vi "NoiseLoop.vi"(8 "error in (no error)":errorcluster, 11 "Queue in":refnum<queue>) -> (0 "error out":errorcluster)   [LabVIEW 2018]
uses:
  Controls/Enums/NoiseQueueElements.ctl
  Controls/Clusts/Noise_Loop_Clust.ctl
  Controls/Clusts/FPGA_Config_Clust.ctl
  Controls/Enums/TargetNumber.ctl
  Controls/Clusts/Config_Clust.ctl
  Controls/Clusts/UserConfig.ctl
  Controls/PathsCluster.ctl
  Controls/Clusts/FrontPanel_UserConfig.ctl
  Controls/Clusts/Inclinometer_User_Cfg.ctl
  Controls/Clusts/FP_UserTargetConfig.ctl
  Controls/Clusts/FreqShift.ctl
  Controls/Clusts/FPGA_Scale.ctl
  Controls/Enums/ScaleMeasure.ctl
  Controls/RadioButtons/FilterEnableRadio.ctl
  Controls/Clusts/AllNoiseData.ctl
  Controls/Clusts/NoiseFloorData.ctl
  Controls/Clusts/Noise_Targets_Initialized.ctl
  Controls/Clusts/FPGA_Probes.ctl
  Controls/Enums/FP_Loop_Enum.ctl
  Controls/Enums/LogLoopEnum.ctl
  HDF5/HDF5_NoiseInfoClust.ctl
  Controls/Enums/WatchdogTimer_Enum.ctl
  <vilib>/Utility/error.llb/Error Cluster From Error Code.vi
  <vilib>/rvi/errors/niLvFpgaAdjustHostInterfaceError.vi
  <vilib>/rvi/interface/nirviMethod/nirviMethod.xnode
  <vilib>/rvi/interface/nirviReadWriteControl/nirviReadWriteControl.xnode
  <vilib>/FPGAPlugInAG/Dynamic/niLvFpga_StartFifo_Dynamic.vi
  <vilib>/rvi/errors/niLvFpgaMergeErrorWithErrorCode.vi
  <vilib>/FPGAPlugInAG/Dynamic/niLvFpga_ReadFifo_Dynamic.vi
  NiFpgaLv.dll
  <vilib>/rvi/interface/Simulation/niFpgaSimulationCallBeginRW.vi
panel:
  out "Elapsed":u32
  out "NoiseLoopCount":i32
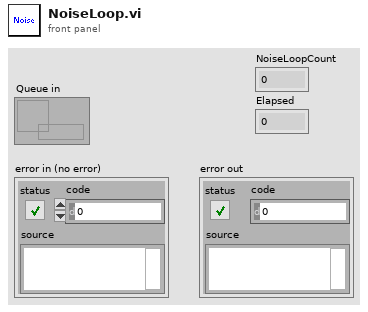
[diagram p1: front panel]
types:
  T1 = typedef "Noise_Loop_Clust.ctl" = cluster{"FPGA":T2, "Config":T4, "AllNoise":T14, "Init'd":T16}
  T2 = typedef "FPGA_Config_Clust.ctl" = cluster{"Target":T3, "Channel":T3, "Ref1":refnum<k20>, "Ref2":refnum<k20>}
  T3 = typedef "TargetNumber.ctl" = enum16{"1", "2", "3", "4"}
  T4 = typedef "Config_Clust.ctl" = cluster{"UsrCfg":T5, "FP_User":T7}
  T5 = typedef "UserConfig.ctl" = cluster{"Paths":T6, "SampleRate":dbl}
  T6 = typedef "PathsCluster.ctl" = cluster{"CfgFile":path, "LogFolder":path, "LogFile":path, "NAS path":path, "ThreshFile":path, "RedunFolder":path}
  T7 = typedef "FrontPanel_UserConfig.ctl" = cluster{"#NoiseSums":u32, "Max_df":u32, "AvgAvg":bool, "#Avg":u16, "AutoCenter":bool, "Inclin":T8, "1":T9, "2":T9, "3":T9, "4":T9, "Target to Probe":T3, "SNR_Thresh":dbl, "Paths":T6, "Connex_Location":string, "SimulateFPGA":bool, "Deadband":dbl}
  T8 = typedef "Inclinometer_User_Cfg.ctl" = cluster{"Vmin":dbl, "Vmax":dbl, "Angle_min":dbl, "Angle_max":dbl, "Offset":dbl, "Pos_Neg":bool}
  T9 = typedef "FP_UserTargetConfig.ctl" = cluster{"Cal_":T10, "Beac":T10, "Scale":T11, "Offset":fxp<+/-,16,16>, "Scale_Noise":fxp<+/-,30,30>, "Scale_Step1":fxp<+/-,17,17>, "Scale_In_RT":ext, "ScaleMeas":fxp<+/-,16,1>, "FreqsToRemove":i32[], "Width":i32[], "ScaleMeasEnum":T12, "FilterEnab":T13}
  T10 = typedef "FreqShift.ctl" = cluster{"Fine":dbl, "Coarse_":dbl}
  T11 = typedef "FPGA_Scale.ctl" = cluster{"Step4":fxp<+/-,23,23>, "Step5":fxp<+/-,23,23>, "Step6":fxp<+/-,23,23>, "Step7":fxp<+/-,23,23>}
  T12 = typedef "ScaleMeasure.ctl" = enum16{"1", "10", "50", "42"}
  T13 = typedef "FilterEnableRadio.ctl" = enum32{"None", "Step 1", "Frequency Shift", "Step 4", "Step 5", "Step 6", "Step 7"}
  T14 = typedef "AllNoiseData.ctl" = cluster{"1":T15, "2":T15, "3":T15, "4":T15}
  T15 = typedef "NoiseFloorData.ctl" = cluster{"df":dbl, "AvgAvgSpectrum":dbl[], "FFT_Index":i32[], "Avg'd":dbl[], "Sum":dbl, "SumdSpectrum":dbl[], "SumCount":u32, "DayOfYear":i32}
  T16 = typedef "Noise_Targets_Initialized.ctl" = cluster{"1":bool, "2":bool, "3":bool, "4":bool}
  T17 = typedef "NoiseQueueElements.ctl" = enum16{"Noise_Startup", "Noise_Init", "Noise_Macro", "Noise_Config", "Noise_NewData", "Noise_Transform", "Noise_SumdTrace", "Noise_Send", "Noise_Probes", "Noise_Exit"}
  T18 = typedef "FPGA_Probes.ctl" = cluster{"Probe 1":i16, "Probe 2":fxp<+/-,16,16>, "Probe 3":fxp<+/-,39,24>, "Probe 4":fxp<+/-,39,24>, "Probe 5":fxp<+/-,16,2>, "Probe 6":fxp<+/-,33,19>, "Probe 7":fxp<+/-,18,1>, "Probe 7_1":fxp<+/-,18,1>, "IProbe":cluster{"Probe 8":fxp<+/-,18,1>, "Probe 9":fxp<+/-,24,1>, "Probe 10":fxp<+/-,24,1>, "Probe 11":fxp<+/-,24,1>, "Probe 12":fxp<+/-,47,24>, "Probe 13":fxp<+/-,24,1>, "Probe 14":fxp<+/-,25,2>, "Probe 15":fxp<+/-,48,25>, "Probe 16":fxp<+/-,24,1>, "Probe 17":fxp<+/-,25,2>, "Probe 18":fxp<+/-,48,25>, "Probe 19":fxp<+/-,24,1>, "Probe20":fxp<+/-,24,1>}, "Probe 21":fxp<+/-,24,5>, "Probe 22":fxp<+/-,54,35>, "Probe 23":fxp<+/-,54,1>, "Probe 24":fxp<+/-,16,1>, "Probe Offsetd":fxp<+/-,16,16>, "CalShiftProbe":fxp<+/-,48,0>, "QProbe":cluster{"Probe 8":fxp<+/-,18,1>, "Probe 9":fxp<+/-,24,1>, "Probe 10":fxp<+/-,24,1>, "Probe 11":fxp<+/-,24,1>, "Probe 12":fxp<+/-,47,24>, "Probe 13":fxp<+/-,24,1>, "Probe 14":fxp<+/-,25,2>, "Probe 15":fxp<+/-,48,25>, "Probe 16":fxp<+/-,24,1>, "Probe 17":fxp<+/-,25,2>, "Probe 18":fxp<+/-,48,25>, "Probe 19":fxp<+/-,24,1>, "Probe20":fxp<+/-,24,1>}, "AI_Over":bool, "10MHzLocked":bool}
  T19 = typedef "LogLoopEnum.ctl" = enum16{"Log_Init", "Log_Config", "Log_CfgAlarm", "Log_TimeDomain", "Log_Tone", "Log_NoiseTrace", "Log_NoiseSum", "Log_DO", "Log_AI", "Log_TC", "Log_Disdrom", "Log_Weather", "Log_TE", "Log_ADAM", "Log_UPS", "Log_ChkTime", "Log_Alarm", "Log_SSH", "Log_Write", "Log_Exit"}
  T20 = typedef "WatchdogTimer_Enum.ctl" = enum16{"ResetAll", "CheckAll", "HW1", "HW2", "Tones", "FP", "Noise", "Log", "TCP", "AI", "TC", "ADAM", "Disdrom", "TE", "Weather"}
  T21 = typedef "HDF5_NoiseInfoClust.ctl" = cluster{"Timestring":string, "Timestamp":dbl, "df":dbl, "Sum":dbl}
  T22 = typedef "FP_Loop_Enum.ctl" = enum16{"FP_Init", "FP_Scale", "FP_Tone", "FP_Noise", "FP_Probes", "FP_PXI", "FP_AI", "FP_TC", "FP_PWR_Hist", "FP_Alarm", "FP_Exit"}
  T23 = typedef "LVDateTimeRec.ctl" = cluster{"fractional second":dbl, "second":i32, "minute":i32, "hour":i32, "day of month":i32, "month":i32, "year":i32, "day of week":i32, "day of year":i32, "DST":i32}
  T24 = cluster{"Probe 8":fxp<+/-,18,1>, "Probe 9":fxp<+/-,24,1>, "Probe 10":fxp<+/-,24,1>, "Probe 11":fxp<+/-,24,1>, "Probe 12":fxp<+/-,47,24>, "Probe 13":fxp<+/-,24,1>, "Probe 14":fxp<+/-,25,2>, "Probe 15":fxp<+/-,48,25>, "Probe 16":fxp<+/-,24,1>, "Probe 17":fxp<+/-,25,2>, "Probe 18":fxp<+/-,48,25>, "Probe 19":fxp<+/-,24,1>, "Probe20":fxp<+/-,24,1>}
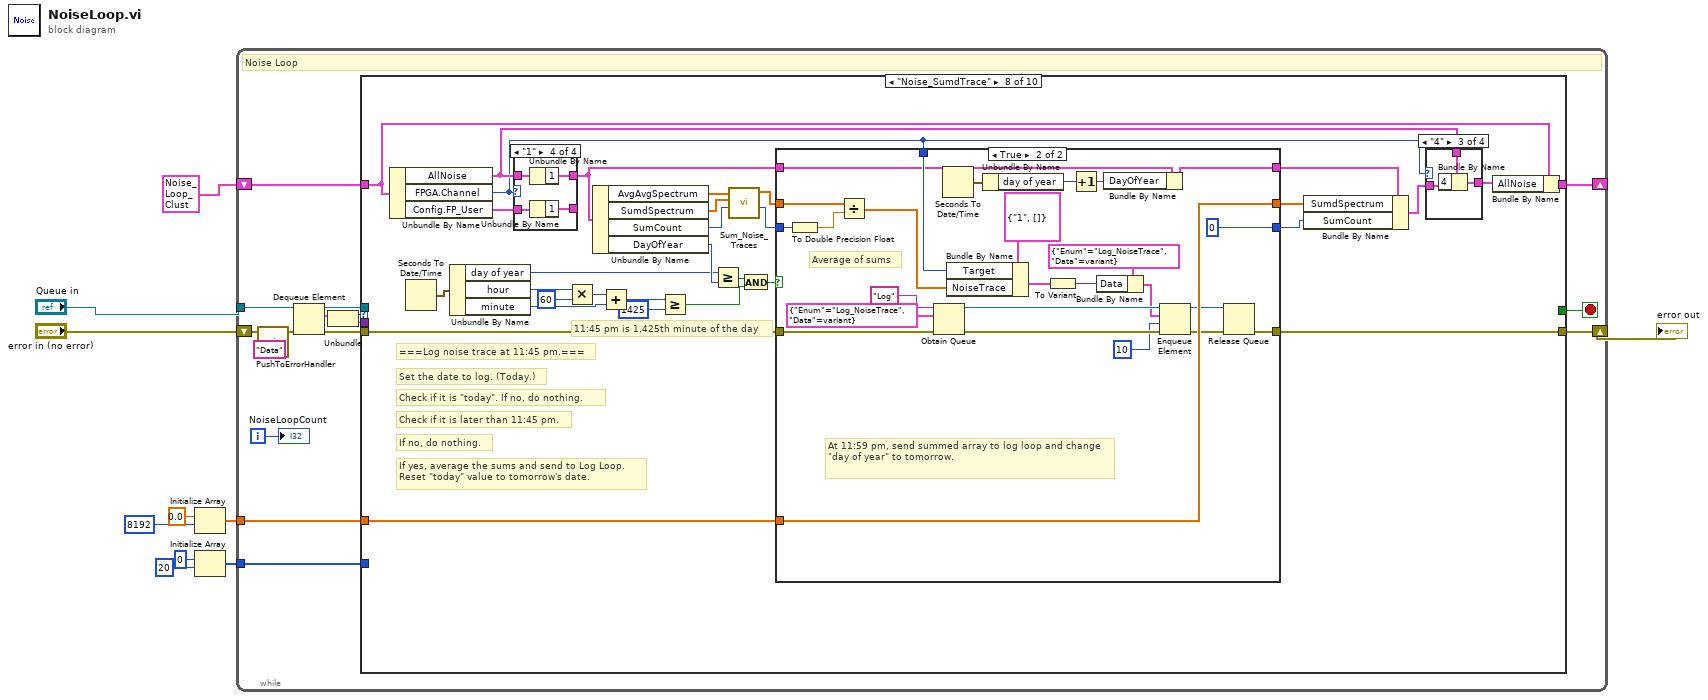
[diagram p0: block diagram]
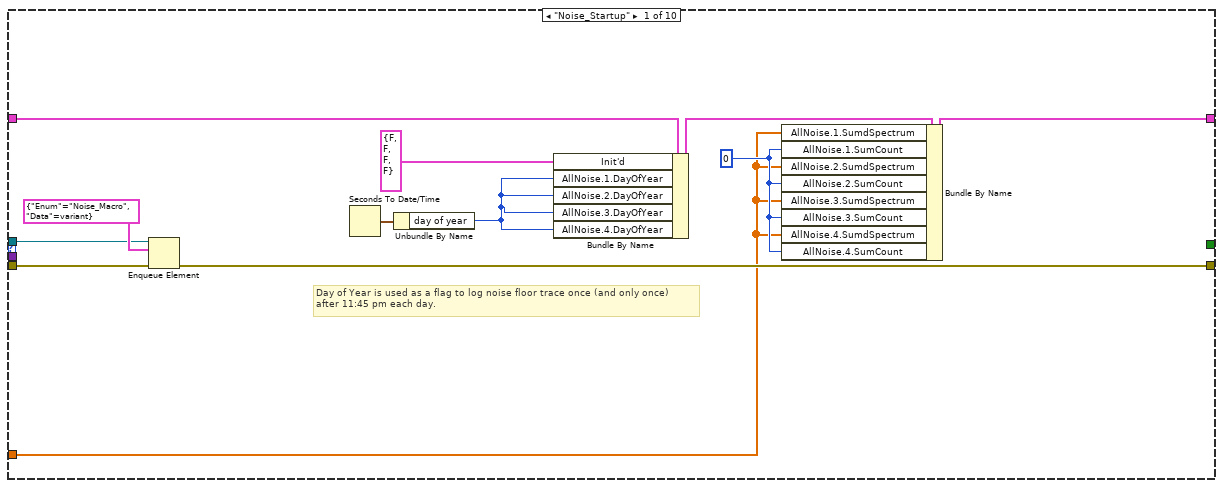
[diagram p2: hidden frame]
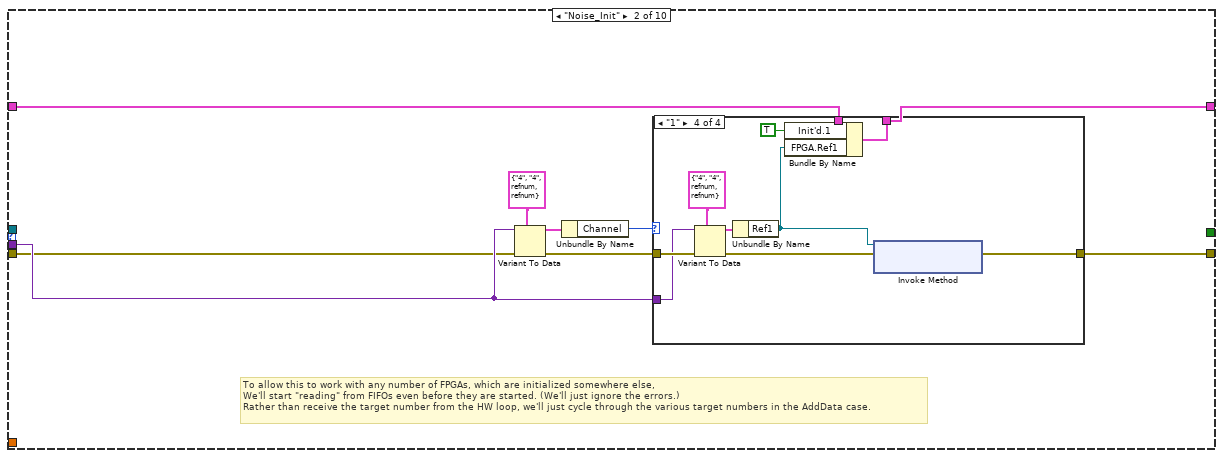
[diagram p3: hidden frame]
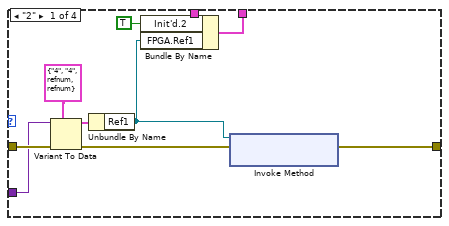
[diagram p4: hidden frame]
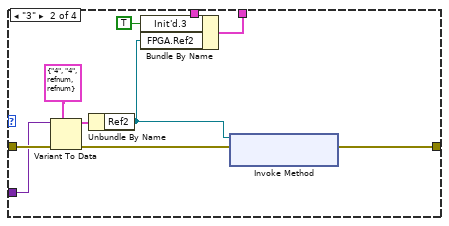
[diagram p5: hidden frame]
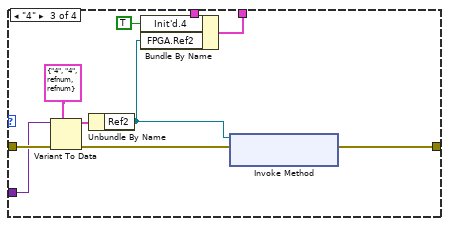
[diagram p6: hidden frame]
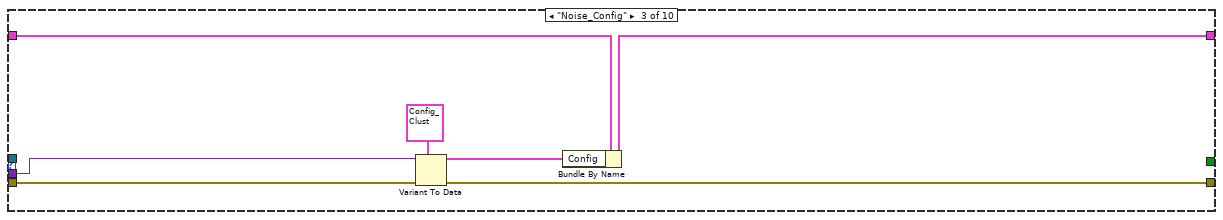
[diagram p7: hidden frame]
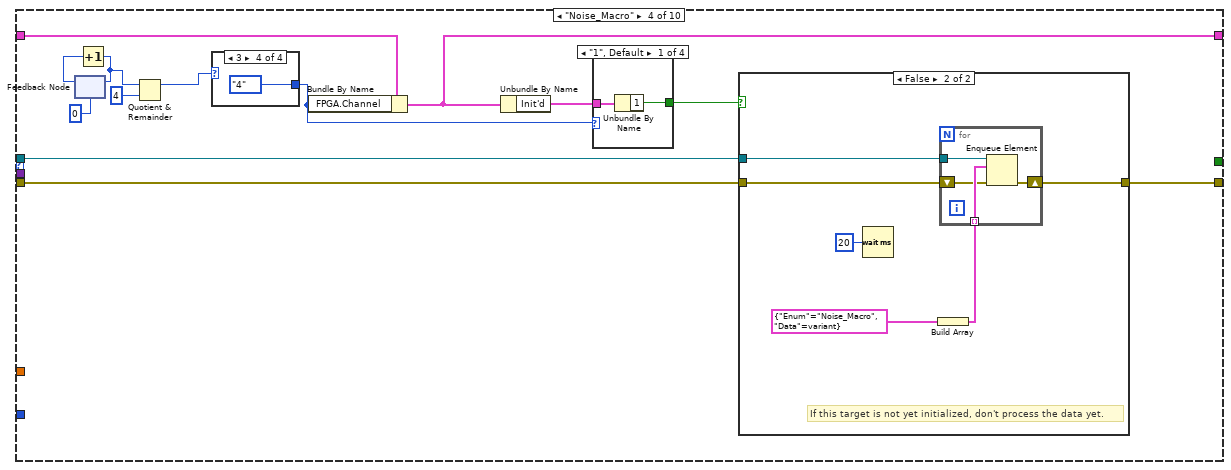
[diagram p8: hidden frame]
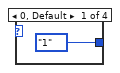
[diagram p9: hidden frame]
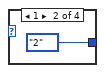
[diagram p10: hidden frame]
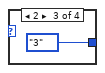
[diagram p11: hidden frame]
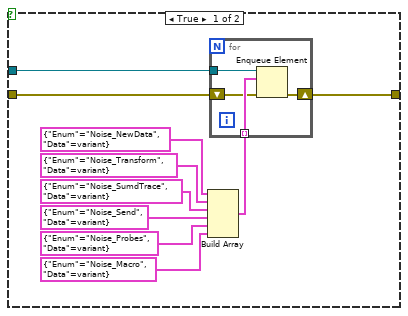
[diagram p12: hidden frame]
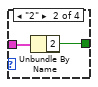
[diagram p13: hidden frame]
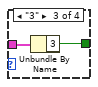
[diagram p14: hidden frame]
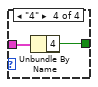
[diagram p15: hidden frame]
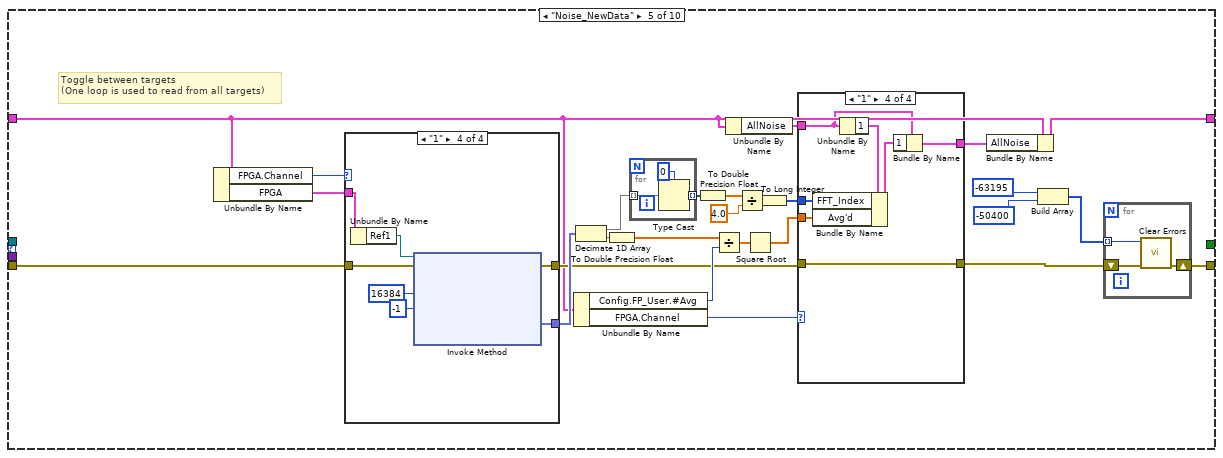
[diagram p16: hidden frame]
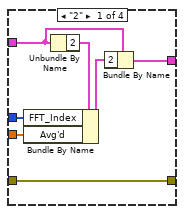
[diagram p17: hidden frame]
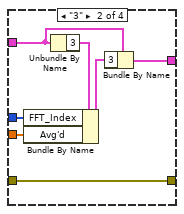
[diagram p18: hidden frame]
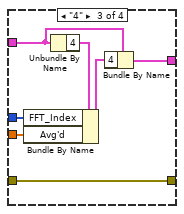
[diagram p19: hidden frame]
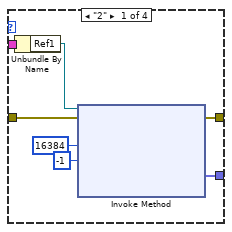
[diagram p20: hidden frame]
diagram:
  n1 = Initialize Array(0.0 ("element"), 8192 ("dimension size")) -> (w5:dbl[])
  n2 = Initialize Array(i16 0 ("element"), 20 ("dimension size")) -> (w8:i16[])
  n3 = while {
    shift-right: [w19] -> w2
    shift-left: "error in (no error)" -> [w24]
    tunnel: "Queue in" -> [w16]
    shift-right: [w14] -> _
    shift-left: T1 {"FPGA"={"Target"=enum."4", "Channel"=enum."4", "Ref1"=refnum, "Ref2"=refnum}, "Config"={"UsrCfg"={"Paths"={"CfgFile"=path "", "LogFolder"=path "", "LogFile"=path "", "NAS path"=path "", "ThreshFile"=path "", "RedunFolder"=path ""}, "SampleRate"=12500.0}, "FP_User"={"#NoiseSums"=1, "Max_df"=1, "AvgAvg"=FALSE, "#Avg"=1, "AutoCenter"=FALSE, "Inclin"={"Vmin"=0.0, "Vmax"=0.0, "Angle_min"=0.0, "Angle_max"=0.0, "Offset"=0.0, "Pos_Neg"=FALSE}, "1"={"Cal_"={"Fine"=0.000213623046875, "Coarse_"=4194303.0}, "Beac"={"Fine"=4194303.0, "Coarse_"=1.0}, "Scale"={"Step4"=10000.0, "Step5"=4194303.0, "Step6"=1.0, "Step7"=10000.0}, "Offset"=0.0, "Scale_Noise"=4194303.0, "Scale_Step1"=65535.0, "Scale_In_RT"=1.0, "ScaleMeas"=0.999969482421875, "FreqsToRemove"=[0, 1633], "Width"=[0, 1633], "ScaleMeasEnum"=enum."50", "FilterEnab"=enum."Step 1"}, "2"={"Cal_"={"Fine"=0.000213623046875, "Coarse_"=4194303.0}, "Beac"={"Fine"=0.000213623046875, "Coarse_"=4194303.0}, "Scale"={"Step4"=0.0, "Step5"=4194303.0, "Step6"=1.0, "Step7"=10000.0}, "Offset"=0.0, "Scale_Noise"=4194303.0, "Scale_Step1"=65535.0, "Scale_In_RT"=1.0, "ScaleMeas"=0.999969482421875, "FreqsToRemove"=[0, 1633], "Width"=[0, 1633], "ScaleMeasEnum"=enum."50", "FilterEnab"=enum."Step 1"}, "3"={"Cal_"={"Fine"=0.000213623046875, "Coarse_"=4194303.0}, "Beac"={"Fine"=0.000213623046875, "Coarse_"=4194303.0}, "Scale"={"Step4"=0.0, "Step5"=4194303.0, "Step6"=1.0, "Step7"=10000.0}, "Offset"=0.0, "Scale_Noise"=4194303.0, "Scale_Step1"=65535.0, "Scale_In_RT"=1.0, "ScaleMeas"=0.999969482421875, "FreqsToRemove"=[0, 1633], "Width"=[0, 1633], "ScaleMeasEnum"=enum."50", "FilterEnab"=enum."Step 1"}, "4"={"Cal_"={"Fine"=0.000213623046875, "Coarse_"=4194303.0}, "Beac"={"Fine"=0.000213623046875, "Coarse_"=4194303.0}, "Scale"={"Step4"=0.0, "Step5"=4194303.0, "Step6"=1.0, "Step7"=10000.0}, "Offset"=0.0, "Scale_Noise"=4194303.0, "Scale_Step1"=1.0, "Scale_In_RT"=10000.0, "ScaleMeas"=0.999969482421875, "FreqsToRemove"=[0, 1633], "Width"=[0, 1633], "ScaleMeasEnum"=enum."50", "FilterEnab"=enum."Step 1"}, "Target to Probe"=enum."4", "SNR_Thresh"=1.0, "Paths"={"CfgFile"=path "", "LogFolder"=path "", "LogFile"=path "", "NAS path"=path "", "ThreshFile"=path "", "RedunFolder"=path ""}, "Connex_Location"="", "SimulateFPGA"=FALSE, "Deadband"=0.0}}, "AllNoise"={"1"={"df"=7629.39453125, "AvgAvgSpectrum"=[], "FFT_Index"=[], "Avg'd"=[], "Sum"=0.0, "SumdSpectrum"=[], "SumCount"=0, "DayOfYear"=0}, "2"={"df"=7629.39453125, "AvgAvgSpectrum"=[], "FFT_Index"=[], "Avg'd"=[], "Sum"=0.0, "SumdSpectrum"=[], "SumCount"=0, "DayOfYear"=0}, "3"={"df"=7629.39453125, "AvgAvgSpectrum"=[], "FFT_Index"=[], "Avg'd"=[], "Sum"=0.0, "SumdSpectrum"=[], "SumCount"=0, "DayOfYear"=0}, "4"={"df"=7629.39453125, "AvgAvgSpectrum"=[], "FFT_Index"=[], "Avg'd"=[], "Sum"=0.0, "SumdSpectrum"=[], "SumCount"=0, "DayOfYear"=0}}, "Init'd"={"1"=FALSE, "2"=FALSE, "3"=FALSE, "4"=FALSE}} -> [w15]
    tunnel: w5 -> [w13]
    tunnel: w8 -> [w12]
    i -> [w11]
    stop <- w17 stop-if-true
    # "Noise Loop"
    n4 = call "PushToErrorHandler.vi"("ErrorIn"=w24, "ErrorLocation"="Data") -> ("ErrorOut"=w23:errorcluster)  [unwired: 5 in]
    n5 = Dequeue Element(queue=w16, error in (no error)=w23) -> (queue out=w18:refnum<queue>, element=w26:cluster{"Enum":T17, "Data":variant}, error out=w20:errorcluster)  [unwired: 1 in, 1 out]
    n6 = Unbundle(w26) -> ("Enum"=w25:T17, "Data"=w21:variant)
    n7 = case shown="\"Noise_SumdTrace\"" w25 {
      tunnel: w21 -> [_ w42 w93 _ _ _ _ _ _ _]
      tunnel: w20 -> [w34 w39 w92 w106 w147 w266 w371 w445 w512 w581]
      tunnel: [w33 w47 w94 w105 w161 w264 w370 w444 w528 w582] -> w19
      tunnel: w18 -> [w31 _ _ w107 _ _ _ _ _ w580]
      tunnel: [_ _ _ _ _ _ _ _ _ TRUE] -> w17
      tunnel: [w29 w43 w90 w103 w155 w263 w360 w448 w540 w578] -> w14
      tunnel: w15 -> [w38 w40 w91 w104 w146 w263 w367 w452 w540 w578]
      tunnel: w13 -> [w32 _ _ _ _ _ w359 w438 _ _]
      tunnel: w12 -> [_ _ _ _ _ w265 _ _ _ _]
      frame "Noise_Startup" {
        w35 = u32 0 ("AllNoise.1.SumCount")
        # "Day of Year is used as a flag to log noise floor trace once (and only once)\nafter 11:45 pm each day."
        n8 = Enqueue Element(queue=w31, element=cluster{"Enum":T17, "Data":variant} {"Enum"=enum."Noise_Macro", "Data"=variant}, error in (no error)=w34) -> (error out=w33:errorcluster)  [unwired: 1 in, 2 out]
        n9 = Seconds To Date/Time() -> (date time rec=w28:T23)  [unwired: 2 in]
        n10 = Unbundle By Name(w28) -> ("day of year"=w27:i32)
        n11 = Bundle By Name(cluster=w38, "Init'd"=T16 {"1"=FALSE, "2"=FALSE, "3"=FALSE, "4"=FALSE}, "AllNoise.1.DayOfYear"=w27, "AllNoise.2.DayOfYear"=w27, "AllNoise.3.DayOfYear"=w27, "AllNoise.4.DayOfYear"=w27) -> (w30:T1)
        n12 = Bundle By Name(cluster=w30, "AllNoise.1.SumdSpectrum"=w32, "AllNoise.1.SumCount"=w35, "AllNoise.2.SumdSpectrum"=w32, "AllNoise.2.SumCount"=w35, "AllNoise.3.SumdSpectrum"=w32, "AllNoise.3.SumCount"=w35, "AllNoise.4.SumdSpectrum"=w32, "AllNoise.4.SumCount"=w35) -> (w29:T1)
      }
      frame "Noise_Init" {
        # "To allow this to work with any number of FPGAs, which are initialized somewhere else,\nWe'll start \"reading\" from FIFOs even before they are started. (We'll just ignore the errors.)\nRather than receive the target number from the HW loop, we'll just cycle through the various target numbers in the AddData case."
        n13 = Variant To Data(error in=w39, type=T2 {"Target"=enum."4", "Channel"=enum."4", "Ref1"=refnum, "Ref2"=refnum} ("FPGA"), Variant=w42) -> (data=w44:T2, error out=w45:errorcluster)
        n14 = Unbundle By Name(w44) -> ("Channel"=w41:T3)
        n15 = case shown="\"1\"" w41 {
          tunnel: [w57 w67 w77 w87] -> w47
          tunnel: w45 -> [w55 w65 w75 w85]
          tunnel: w40 -> [w52 w62 w72 w82]
          tunnel: [w51 w61 w71 w81] -> w43
          tunnel: w42 -> [w49 w59 w69 w79]
          frame "2" {
            n16 = Variant To Data(error in=w55, type=T2 {"Target"=enum."4", "Channel"=enum."4", "Ref1"=refnum, "Ref2"=refnum} ("FPGA"), Variant=w49) -> (data=w53:T2, error out=w54:errorcluster)
            n17 = Unbundle By Name(w53) -> ("Ref1"=w50:refnum<k20>)
            n18 = Bundle By Name(cluster=w52, "Init'd.2"=TRUE, "FPGA.Ref1"=w50) -> (w51:T1)
            n19 = xnode "Invoke Method"("FPGA VI Reference In"=w50, "error in"=w54) -> ("error out"=w57:errorcluster)  [unwired: 1 out]
          }
          frame "3" {
            n20 = Variant To Data(error in=w65, type=T2 {"Target"=enum."4", "Channel"=enum."4", "Ref1"=refnum, "Ref2"=refnum} ("FPGA"), Variant=w59) -> (data=w63:T2, error out=w64:errorcluster)
            n21 = Unbundle By Name(w63) -> ("Ref2"=w60:refnum<k20>)
            n22 = Bundle By Name(cluster=w62, "Init'd.3"=TRUE, "FPGA.Ref2"=w60) -> (w61:T1)
            n23 = xnode "Invoke Method"("FPGA VI Reference In"=w60, "error in"=w64) -> ("error out"=w67:errorcluster)  [unwired: 1 out]
          }
          frame "4" {
            n24 = Variant To Data(error in=w75, type=T2 {"Target"=enum."4", "Channel"=enum."4", "Ref1"=refnum, "Ref2"=refnum} ("FPGA"), Variant=w69) -> (data=w73:T2, error out=w74:errorcluster)
            n25 = Unbundle By Name(w73) -> ("Ref2"=w70:refnum<k20>)
            n26 = Bundle By Name(cluster=w72, "Init'd.4"=TRUE, "FPGA.Ref2"=w70) -> (w71:T1)
            n27 = xnode "Invoke Method"("FPGA VI Reference In"=w70, "error in"=w74) -> ("error out"=w77:errorcluster)  [unwired: 1 out]
          }
          frame "1" {
            n28 = Variant To Data(error in=w85, type=T2 {"Target"=enum."4", "Channel"=enum."4", "Ref1"=refnum, "Ref2"=refnum} ("FPGA"), Variant=w79) -> (data=w83:T2, error out=w84:errorcluster)
            n29 = Unbundle By Name(w83) -> ("Ref1"=w80:refnum<k20>)
            n30 = Bundle By Name(cluster=w82, "Init'd.1"=TRUE, "FPGA.Ref1"=w80) -> (w81:T1)
            n31 = xnode "Invoke Method"("FPGA VI Reference In"=w80, "error in"=w84) -> ("error out"=w87:errorcluster)  [unwired: 1 out]
          }
        }
      }
      frame "Noise_Config" {
        n32 = Variant To Data(error in=w92, type=T4 {"UsrCfg"={"Paths"={"CfgFile"=path "", "LogFolder"=path "", "LogFile"=path "", "NAS path"=path "", "ThreshFile"=path "", "RedunFolder"=path ""}, "SampleRate"=12500.0}, "FP_User"={"#NoiseSums"=1, "Max_df"=1, "AvgAvg"=FALSE, "#Avg"=1, "AutoCenter"=FALSE, "Inclin"={"Vmin"=0.0, "Vmax"=0.0, "Angle_min"=0.0, "Angle_max"=0.0, "Offset"=0.0, "Pos_Neg"=FALSE}, "1"={"Cal_"={"Fine"=0.000213623046875, "Coarse_"=4194303.0}, "Beac"={"Fine"=4194303.0, "Coarse_"=1.0}, "Scale"={"Step4"=10000.0, "Step5"=4194303.0, "Step6"=1.0, "Step7"=10000.0}, "Offset"=0.0, "Scale_Noise"=4194303.0, "Scale_Step1"=65535.0, "Scale_In_RT"=1.0, "ScaleMeas"=0.999969482421875, "FreqsToRemove"=[0, 1633], "Width"=[0, 1633], "ScaleMeasEnum"=enum."50", "FilterEnab"=enum."Step 1"}, "2"={"Cal_"={"Fine"=0.000213623046875, "Coarse_"=4194303.0}, "Beac"={"Fine"=0.000213623046875, "Coarse_"=4194303.0}, "Scale"={"Step4"=0.0, "Step5"=4194303.0, "Step6"=1.0, "Step7"=10000.0}, "Offset"=0.0, "Scale_Noise"=4194303.0, "Scale_Step1"=65535.0, "Scale_In_RT"=1.0, "ScaleMeas"=0.999969482421875, "FreqsToRemove"=[0, 1633], "Width"=[0, 1633], "ScaleMeasEnum"=enum."50", "FilterEnab"=enum."Step 1"}, "3"={"Cal_"={"Fine"=0.000213623046875, "Coarse_"=4194303.0}, "Beac"={"Fine"=0.000213623046875, "Coarse_"=4194303.0}, "Scale"={"Step4"=0.0, "Step5"=4194303.0, "Step6"=1.0, "Step7"=10000.0}, "Offset"=0.0, "Scale_Noise"=4194303.0, "Scale_Step1"=65535.0, "Scale_In_RT"=1.0, "ScaleMeas"=0.999969482421875, "FreqsToRemove"=[0, 1633], "Width"=[0, 1633], "ScaleMeasEnum"=enum."50", "FilterEnab"=enum."Step 1"}, "4"={"Cal_"={"Fine"=0.000213623046875, "Coarse_"=4194303.0}, "Beac"={"Fine"=0.000213623046875, "Coarse_"=4194303.0}, "Scale"={"Step4"=0.0, "Step5"=4194303.0, "Step6"=1.0, "Step7"=10000.0}, "Offset"=0.0, "Scale_Noise"=4194303.0, "Scale_Step1"=1.0, "Scale_In_RT"=10000.0, "ScaleMeas"=0.999969482421875, "FreqsToRemove"=[0, 1633], "Width"=[0, 1633], "ScaleMeasEnum"=enum."50", "FilterEnab"=enum."Step 1"}, "Target to Probe"=enum."4", "SNR_Thresh"=1.0, "Paths"={"CfgFile"=path "", "LogFolder"=path "", "LogFile"=path "", "NAS path"=path "", "ThreshFile"=path "", "RedunFolder"=path ""}, "Connex_Location"="", "SimulateFPGA"=FALSE, "Deadband"=0.0}} ("Config"), Variant=w93) -> (data=w88:T4, error out=w94:errorcluster)
        n33 = Bundle By Name(cluster=w91, "Config"=w88) -> (w90:T1)
      }
      frame "Noise_Macro" {
        n34 = feedback #1(0) -> (w99:i32)
        n35 = Increment(x=w99) -> (x+1=w97:i32)
        n36 = feedback-in #1(w97) -> ()
        n37 = Quotient & Remainder(x=w97, y=4) -> (x-y*floor(x/y)=w95:i32)  [unwired: 1 out]
        n38 = case shown="3" w95 {
          tunnel: [TargetNumber."1" ("FPGA.Target") TargetNumber."2" ("FPGA.Target") TargetNumber."3" ("FPGA.Target") TargetNumber."4" ("FPGA.Target")] -> w98
          frame 0, Default {
          }
          frame 1 {
          }
          frame 2 {
          }
          frame 3 {
          }
        }
        n39 = Bundle By Name(cluster=w104, "FPGA.Channel"=w98) -> (w103:T1)
        n40 = Unbundle By Name(w103) -> ("Init'd"=w102:T16)
        n41 = case shown="\"1\", Default" w98 {
          tunnel: w102 -> [w137 w139 w141 w143]
          tunnel: [w136 w138 w140 w142] -> w101
          frame "1", Default {
            n42 = Unbundle By Name(w137) -> ("1"=w136:bool)
          }
          frame "2" {
            n43 = Unbundle By Name(w139) -> ("2"=w138:bool)
          }
          frame "3" {
            n44 = Unbundle By Name(w141) -> ("3"=w140:bool)
          }
          frame "4" {
            n45 = Unbundle By Name(w143) -> ("4"=w142:bool)
          }
        }
        n46 = case shown="False" w101 {
          tunnel: w107 -> [w119 w130]
          tunnel: w106 -> [w117 w129]
          tunnel: [w114 w128] -> w105
          frame True {
            n47 = Build Array(cluster{"Enum":T17, "Data":variant} {"Enum"=enum."Noise_NewData", "Data"=variant} ("element"), cluster{"Enum":T17, "Data":variant} {"Enum"=enum."Noise_Transform", "Data"=variant} ("element"), cluster{"Enum":T17, "Data":variant} {"Enum"=enum."Noise_SumdTrace", "Data"=variant} ("element"), cluster{"Enum":T17, "Data":variant} {"Enum"=enum."Noise_Send", "Data"=variant} ("element"), cluster{"Enum":T17, "Data":variant} {"Enum"=enum."Noise_Probes", "Data"=variant} ("element"), cluster{"Enum":T17, "Data":variant} {"Enum"=enum."Noise_Macro", "Data"=variant} ("element")) -> (w121:cluster{"Enum":T17, "Data":variant}[])
            n48 = for {
              tunnel: w121 -> [w125] mode=indexing
              tunnel: w119 -> [w122]
              shift-right: [w123] -> w114
              shift-left: w117 -> [w124]
              n49 = Enqueue Element(queue=w122, element=w125, error in (no error)=w124) -> (error out=w123:errorcluster)  [unwired: 1 in, 2 out]
            }
          }
          frame False {
            # "If this target is not yet initialized, don't process the data yet."
            n50 = Wait (ms)(milliseconds to wait=u32 20) -> ()  [unwired: 1 out]
            n51 = Build Array(cluster{"Enum":T17, "Data":variant} {"Enum"=enum."Noise_Macro", "Data"=variant} ("element")) -> (w131:cluster{"Enum":T17, "Data":variant}[])
            n52 = for {
              tunnel: w131 -> [w135] mode=indexing
              tunnel: w130 -> [w132]
              shift-right: [w133] -> w128
              shift-left: w129 -> [w134]
              n53 = Enqueue Element(queue=w132, element=w135, error in (no error)=w134) -> (error out=w133:errorcluster)  [unwired: 1 in, 2 out]
            }
          }
        }
      }
      frame "Noise_NewData" {
        # "Toggle between targets\n(One loop is used to read from all targets)"
        n54 = Unbundle By Name(w146) -> ("FPGA.Channel"=w145:T3, "FPGA"=w158:T2)
        n55 = case shown="\"1\"" w145 {
          tunnel: [w207 w209 w221 w228] -> w162
          tunnel: w147 -> [w204 w214 w218 w225]
          tunnel: [w203 w208 w217 w224] -> w152
          tunnel: w158 -> [w201 w213 w215 w222]
          frame "2" {
            n56 = Unbundle By Name(w201) -> ("Ref1"=w202:refnum<k20>)
            n57 = xnode "Invoke Method"("FPGA VI Reference In"=w202, "error in"=w204, "Number of Elements"=u32 16384, "Timeout (ms)"=-1) -> ("error out"=w203:errorcluster, "Data"=w207:fxp<+/-,30,15>[])  [unwired: 2 out]
          }
          frame "3" {
            n58 = Unbundle By Name(w213) -> ("Ref2"=w212:refnum<k20>)
            n59 = xnode "Invoke Method"("FPGA VI Reference In"=w212, "error in"=w214, "Number of Elements"=u32 16384, "Timeout (ms)"=-1) -> ("error out"=w208:errorcluster, "Data"=w209:fxp<+/-,30,15>[])  [unwired: 2 out]
          }
          frame "4" {
            n60 = Unbundle By Name(w215) -> ("Ref2"=w216:refnum<k20>)
            n61 = xnode "Invoke Method"("FPGA VI Reference In"=w216, "error in"=w218, "Number of Elements"=u32 16384, "Timeout (ms)"=-1) -> ("error out"=w217:errorcluster, "Data"=w221:fxp<+/-,30,15>[])  [unwired: 2 out]
          }
          frame "1" {
            n62 = Unbundle By Name(w222) -> ("Ref1"=w223:refnum<k20>)
            n63 = xnode "Invoke Method"("FPGA VI Reference In"=w223, "error in"=w225, "Number of Elements"=u32 16384, "Timeout (ms)"=-1) -> ("error out"=w224:errorcluster, "Data"=w228:fxp<+/-,30,15>[])  [unwired: 2 out]
          }
        }
        n64 = Unbundle By Name(w146) -> ("Config.FP_User.#Avg"=w157:u16, "FPGA.Channel"=w153:T3)
        n65 = Decimate 1D Array(w162) -> (w166:fxp<+/-,30,15>[], w163:fxp<+/-,30,15>[])
        n66 = To Double Precision Float(number=w163) -> (double precision float=w169:dbl[])
        n67 = for {
          tunnel: w166 -> [w230] mode=indexing
          tunnel: [w229] -> w168 mode=indexing
          n68 = Type Cast(type=0, x=w230) -> (*(type *) &x=w229:i32)
        }
        n69 = To Double Precision Float(number=w168) -> (double precision float=w164:dbl[])
        n70 = Divide(x=w169, y=w157) -> (x/y=w159:dbl[])
        n71 = Unbundle By Name(w146) -> ("AllNoise"=w156:T14)
        n72 = Divide(x=w164, y=4.0) -> (x/y=w167:dbl[])
        n73 = Square Root(x=w159) -> (sqrt(x)=w144:dbl[])
        n74 = To Long Integer(number=w167) -> (32bit integer=w160:i32[])
        n75 = case shown="\"1\"" w153 {
          tunnel: w160 -> [w179 w186 w193 w200]
          tunnel: w144 -> [w178 w185 w192 w199]
          tunnel: w156 -> [w176 w183 w190 w197]
          tunnel: [w174 w181 w188 w195] -> w154
          tunnel: [w173 w180 w187 w194] -> w151
          tunnel: w152 -> [w173 w180 w187 w194]
          frame "2" {
            n76 = Unbundle By Name(w176) -> ("2"=w177:T15)
            n77 = Bundle By Name(cluster=w177, "FFT_Index"=w179, "Avg'd"=w178) -> (w175:T15)
            n78 = Bundle By Name(cluster=w176, "2"=w175) -> (w174:T14)
          }
          frame "3" {
            n79 = Unbundle By Name(w183) -> ("3"=w184:T15)
            n80 = Bundle By Name(cluster=w184, "FFT_Index"=w186, "Avg'd"=w185) -> (w182:T15)
            n81 = Bundle By Name(cluster=w183, "3"=w182) -> (w181:T14)
          }
          frame "4" {
            n82 = Unbundle By Name(w190) -> ("4"=w191:T15)
            n83 = Bundle By Name(cluster=w191, "FFT_Index"=w193, "Avg'd"=w192) -> (w189:T15)
            n84 = Bundle By Name(cluster=w190, "4"=w189) -> (w188:T14)
          }
          frame "1" {
            n85 = Unbundle By Name(w197) -> ("1"=w198:T15)
            n86 = Bundle By Name(cluster=w198, "FFT_Index"=w200, "Avg'd"=w199) -> (w196:T15)
            n87 = Bundle By Name(cluster=w197, "1"=w196) -> (w195:T14)
          }
        }
        n88 = Bundle By Name(cluster=w146, "AllNoise"=w154) -> (w155:T1)
        n89 = Build Array(-63195 ("specific error code to clear (0: all)"), -50400 ("specific error code to clear (0: all)")) -> (w148:i32[])
        n90 = for {
          tunnel: w148 -> [w170] mode=indexing
          shift-right: [w172] -> w161
          shift-left: w151 -> [w171]
          n91 = call <vilib>:"Clear Errors.vi"("error in (no error)"=w171, "specific error code to clear (0: all)"=w170) -> ("error out"=w172:errorcluster)  [unwired: 4 in, 1 out]
        }
      }
      frame "Noise_Probes" {
        w248 = cluster{"Enum":T22, "Data":variant} {"Enum"=enum."FP_Probes", "Data"=variant}
        # "If the user selects to probe an FPGA that hasn't been init'd yet (only happens during first few seconds of startup)\nthis error (-63195) will occur. Luke 12-12-2017"
        # "This is a way that autoscaling based on signal amplitude could be implemented.\nNot using now. \nWe'd need a conversion that works for multiple ranges.\nLuke 12-5-2017"
        n92 = Unbundle By Name(w263) -> ("Config.FP_User.Target to Probe"=w262:T3)
        n93 = case shown="\"3\"" w262 {
          tunnel: w263 -> [w290 w308 w326 w344]
          tunnel: w266 -> [w289 w307 w325 w343]
          tunnel: [w288 w306 w324 w342] -> w260
          tunnel: [w287 w305 w323 w341] -> w259
          tunnel: [w286 w304 w322 w340] -> w258
          tunnel: [w285 w303 w321 w339] -> w257
          tunnel: [w284 w302 w320 w338] -> w256
          tunnel: [w283 w301 w319 w337] -> w254
          tunnel: [w282 w300 w318 w336] -> w253
          tunnel: [w281 w299 w317 w335] -> w252
          tunnel: [w277 w295 w313 w331] -> w251
          tunnel: [w280 w298 w316 w334] -> w255
          tunnel: [w279 w297 w315 w333] -> w241
          tunnel: [w275 w293 w312 w329] -> w235
          tunnel: [w276 w294 w311 w330] -> w236
          tunnel: [w274 w292 w310 w328] -> w234
          tunnel: [w273 w291 w309 w327] -> w233
          frame "1", Default {
            n94 = Unbundle By Name(w290) -> ("FPGA.Ref1"=w278:refnum<k20>)
            n95 = xnode "Read/Write Control"("FPGA VI Reference In"=w278, "error in"=w289) -> ("error out"=w279:errorcluster, "Probe 3"=w288:fxp<+/-,16,1>, "Probe 21"=w287:fxp<+/-,24,5>, "Probe 22"=w286:fxp<+/-,54,35>, "Probe 23"=w285:fxp<+/-,54,1>, "Probe 24"=w284:fxp<+/-,16,1>, "Probe 1"=w280:i16, "Probe 2"=w283:fxp<+/-,16,16>, "Probe 5"=w282:fxp<+/-,16,2>, "Probe 7"=w281:fxp<+/-,18,1>, "Chan0_Beac_IProbe"=w277:T24, "Chan0_Beac_QProbe"=w276:T24, "Probe Offsetd"=w275:fxp<+/-,16,16>, "AI0_Over"=w274:bool, "Synthesizer Locked"=w273:bool)  [unwired: 1 out]
          }
          frame "2" {
            n96 = Unbundle By Name(w308) -> ("FPGA.Ref1"=w296:refnum<k20>)
            n97 = xnode "Read/Write Control"("FPGA VI Reference In"=w296, "error in"=w307) -> ("error out"=w297:errorcluster, "Probe 3_2"=w306:fxp<+/-,16,1>, "Probe 21_2"=w305:fxp<+/-,24,5>, "Probe 22_2"=w304:fxp<+/-,54,35>, "Probe 23_2"=w303:fxp<+/-,54,1>, "Probe 24_2"=w302:fxp<+/-,16,1>, "Probe 1_2"=w298:i16, "Probe 2_2"=w301:fxp<+/-,16,16>, "Probe 5_2"=w300:fxp<+/-,16,2>, "Probe 7_2"=w299:fxp<+/-,18,1>, "Chan1_Beac_IProbe"=w295:T24, "Chan1_Beac_QProbe"=w294:T24, "Probe Offsetd 2"=w293:fxp<+/-,16,16>, "AI1_Over"=w292:bool, "Synthesizer Locked"=w291:bool)  [unwired: 1 out]
          }
          frame "3" {
            n98 = Unbundle By Name(w326) -> ("FPGA.Ref2"=w314:refnum<k20>)
            n99 = xnode "Read/Write Control"("FPGA VI Reference In"=w314, "error in"=w325) -> ("error out"=w315:errorcluster, "Probe 3"=w324:fxp<+/-,16,1>, "Probe 21"=w323:fxp<+/-,24,5>, "Probe 22"=w322:fxp<+/-,54,35>, "Probe 23"=w321:fxp<+/-,54,1>, "Probe 24"=w320:fxp<+/-,16,1>, "Probe 1"=w316:i16, "Probe 2"=w319:fxp<+/-,16,16>, "Probe 5"=w318:fxp<+/-,16,2>, "Probe 7"=w317:fxp<+/-,18,1>, "Chan0_Beac_IProbe"=w313:T24, "Chan0_Beac_QProbe"=w311:T24, "Probe Offsetd"=w312:fxp<+/-,16,16>, "AI0_Over"=w310:bool, "Synthesizer Locked"=w309:bool)  [unwired: 1 out]
          }
          frame "4" {
            n100 = Unbundle By Name(w344) -> ("FPGA.Ref2"=w332:refnum<k20>)
            n101 = xnode "Read/Write Control"("FPGA VI Reference In"=w332, "error in"=w343) -> ("error out"=w333:errorcluster, "Probe 3_2"=w342:fxp<+/-,16,1>, "Probe 21_2"=w341:fxp<+/-,24,5>, "Probe 22_2"=w340:fxp<+/-,54,35>, "Probe 23_2"=w339:fxp<+/-,54,1>, "Probe 24_2"=w338:fxp<+/-,16,1>, "Probe 1_2"=w334:i16, "Probe 2_2"=w337:fxp<+/-,16,16>, "Probe 5_2"=w336:fxp<+/-,16,2>, "Probe 7_2"=w335:fxp<+/-,18,1>, "Chan1_Beac_IProbe"=w331:T24, "Chan1_Beac_QProbe"=w330:T24, "Probe Offsetd 2"=w329:fxp<+/-,16,16>, "AI1_Over"=w328:bool, "Synthesizer Locked"=w327:bool)  [unwired: 1 out]
          }
        }
        n102 = call <vilib>:"Clear Errors.vi"("error in (no error)"=w241, "specific error code to clear (0: all)"=-63195) -> ("error out"=w242:errorcluster)  [unwired: 4 in, 1 out]
        n103 = Bundle By Name(cluster=T18 {"Probe 1"=0, "Probe 2"=0.0, "Probe 3"=0.0, "Probe 4"=0.0, "Probe 5"=0.0, "Probe 6"=0.0, "Probe 7"=0.0, "Probe 7_1"=0.0, "IProbe"={"Probe 8"=0.0, "Probe 9"=0.0, "Probe 10"=0.0, "Probe 11"=0.0, "Probe 12"=0.0, "Probe 13"=0.0, "Probe 14"=0.0, "Probe 15"=0.0, "Probe 16"=0.0, "Probe 17"=0.0, "Probe 18"=0.0, "Probe 19"=0.0, "Probe20"=0.0}, "Probe 21"=0.0, "Probe 22"=0.0, "Probe 23"=0.0, "Probe 24"=0.0, "Probe Offsetd"=0.0, "CalShiftProbe"=0.0, "QProbe"={"Probe 8"=0.0, "Probe 9"=0.0, "Probe 10"=0.0, "Probe 11"=0.0, "Probe 12"=0.0, "Probe 13"=0.0, "Probe 14"=0.0, "Probe 15"=0.0, "Probe 16"=0.0, "Probe 17"=0.0, "Probe 18"=0.0, "Probe 19"=0.0, "Probe20"=0.0}, "AI_Over"=FALSE, "10MHzLocked"=FALSE} ("FPGA_Probes"), "Probe 3"=w260, "Probe 21"=w259, "Probe 22"=w258, "Probe 23"=w257, "Probe 24"=w256, "Probe 1"=w255, "Probe 2"=w254, "Probe 5"=w253, "Probe 7"=w252, "IProbe"=w251, "QProbe"=w236, "Probe Offsetd"=w235, "AI_Over"=w234, "10MHzLocked"=w233) -> (w247:T18)
        n104 = To Variant(anything=w247) -> (Variant=w246:variant)
        n105 = Obtain Queue(max queue size (-1, unlimited)=100, name (unnamed)="FP", element data type=w248, error in (no error)=w242) -> (queue out=w245:refnum<queue>, error out=w243:errorcluster)  [unwired: 1 in, 1 out]
        n106 = Bundle By Name(cluster=w248, "Data"=w246) -> (w244:cluster{"Enum":T22, "Data":variant})
        n107 = Enqueue Element(queue=w245, element=w244, timeout in ms (-1)=10, error in (no error)=w243) -> (queue out=w237:refnum<queue>, error out=w239:errorcluster)  [unwired: 1 out]
        n108 = Release Queue(queue=w237, error in (no error)=w239) -> (error out=w238:errorcluster)  [unwired: 1 in, 2 out]
        n109 = disable-structure shown="Enabled" {
          disable-tunnel: w265 -> [w271 _]
          disable-tunnel: [w269 w272] -> w264
          disable-tunnel: w255 -> [w268 _]
          disable-tunnel: w238 -> [w267 w272]
          frame Disabled {
            n110 = call "AutoScaleAmplitude.vi"("error in (no error)"=w267, "AutoScale"=FALSE, "Array"=w271, "Probe 1"=w268) -> ("error out"=w269:errorcluster)  [unwired: 7 in]
          }
          frame Enabled {
          }
        }
      }
      frame "Noise_Transform" {
        n111 = Unbundle By Name(w367) -> ("AllNoise"=w365:T14, "FPGA.Channel"=w356:T3, "Config.FP_User"=w369:T7, "Config.FP_User.AvgAvg"=w358:bool)
        n112 = case shown="\"1\"" w356 {
          tunnel: w365 -> [w402 w406 w410 w414]
          tunnel: [w401 w405 w409 w413] -> w364
          tunnel: w369 -> [w400 w404 w408 w412]
          tunnel: [w399 w403 w407 w411] -> w349
          frame "4" {
            n113 = Unbundle By Name(w402) -> ("4"=w401:T15)
            n114 = Unbundle By Name(w400) -> ("4"=w399:T9)
          }
          frame "3" {
            n115 = Unbundle By Name(w406) -> ("3"=w405:T15)
            n116 = Unbundle By Name(w404) -> ("3"=w403:T9)
          }
          frame "2" {
            n117 = Unbundle By Name(w410) -> ("2"=w409:T15)
            n118 = Unbundle By Name(w408) -> ("2"=w407:T9)
          }
          frame "1" {
            n119 = Unbundle By Name(w414) -> ("1"=w413:T15)
            n120 = Unbundle By Name(w412) -> ("1"=w411:T9)
          }
        }
        n121 = Unbundle By Name(w364) -> ("FFT_Index"=w372:i32[], "Avg'd"=w351:dbl[])
        n122 = Unbundle By Name(w349) -> ("FreqsToRemove"=w368:i32[], "Width"=w348:i32[])  [unwired: 1 out]
        n123 = call "Scale_Noise_floor_to_Volts.vi"("1"=w349, "spectrum in"=w351) -> ("Volts"=w350:dbl[])  [unwired: 9 in]
        n124 = for {
          tunnel: w372 -> [w421] mode=indexing
          shift-right: [w419] -> w375
          shift-left: w359 -> [w420]
          shift-right: [w417] -> w374
          shift-left: w359 -> [w418]
          tunnel: w350 -> [w416] mode=indexing
          tunnel: 0.0 ("number") -> [w415]
          n125 = Replace Array Subset(array=w420, new element=w416, index=w421) -> (w419:dbl[])
          n126 = Replace Array Subset(array=w418, new element=w415, index=w421) -> (w417:dbl[])
        }
        n127 = call "FFT To Spectrum_modified_20190812.vi"("real FFT data"=w375, "imaginary FFT data"=w374, "sample rate (S/s)"=125000000.0, "error in (no error)"=w371) -> ("spectrum out (V)"=w355:dbl[], "df (Hz)"=w345:dbl, "error out"=w370:errorcluster)  [unwired: 8 in, 1 out]
        n128 = To Double Precision Float(number=w348) -> (double precision float=w347:dbl[])
        n129 = call "RemoveZeros.vi"("spectrum in"=w355) -> ("Spectrum"=w354:dbl[])  [unwired: 10 in]
        n130 = case shown="\"1\", Default" w356 {
          tunnel: [w377 w382 w384 w386] -> w352
          tunnel: w354 -> [w376 w381 w383 w385]
          frame "2" {
            n131 = call "AverageOfAverageNoiseFloor.vi"("spectrum in"=w376) -> ("AveragedSpectrum"=w377:dbl[])  [unwired: 10 in]
          }
          frame "1", Default {
            n132 = Tick Count (ms)() -> (millisecond timer value=w378:u32)
            n133 = feedback #2() -> (w379:u32)  [unwired: 1 in]
            n134 = feedback-in #2(w378) -> ()
            n135 = call "AverageOfAverageNoiseFloor.vi"("spectrum in"=w381) -> ("AveragedSpectrum"=w382:dbl[])  [unwired: 10 in]
            n136 = Subtract(x=w378, y=w379) -> (x-y=→"Elapsed":u32)
          }
          frame "3" {
            n137 = call "AverageOfAverageNoiseFloor.vi"("spectrum in"=w383) -> ("AveragedSpectrum"=w384:dbl[])  [unwired: 10 in]
          }
          frame "4" {
            n138 = call "AverageOfAverageNoiseFloor.vi"("spectrum in"=w385) -> ("AveragedSpectrum"=w386:dbl[])  [unwired: 10 in]
          }
        }
        n139 = To Double Precision Float(number=w368) -> (double precision float=w346:dbl[])
        n140 = Select(t=w352, s=w358, f=w354) -> (s? t:f=w357:dbl[])
        n141 = call "Scale_Noise_floor_to_dBm.vi"("spectrum in (Volts)"=w357) -> ("Spectrum_dBm"=w353:dbl[])  [unwired: 10 in]
        n142 = call "SumNoiseFloor.vi"("df"=w345, "Width [bins]"=w347, "frequencies to remove [Hz]"=w346, "Spectrum_dBm"=w353) -> ("Numeric"=w362:dbl)  [unwired: 7 in]
        n143 = Bundle By Name(cluster=w364, "AvgAvgSpectrum"=w353, "df"=w345, "Sum"=w362) -> (w366:T15)
        n144 = case shown="\"4\"" w356 {
          tunnel: w366 -> [w389 w392 w395 w398]
          tunnel: w365 -> [w388 w391 w394 w397]
          tunnel: [w387 w390 w393 w396] -> w363
          frame "2" {
            n145 = Bundle By Name(cluster=w388, "2"=w389) -> (w387:T14)
          }
          frame "3" {
            n146 = Bundle By Name(cluster=w391, "3"=w392) -> (w390:T14)
          }
          frame "4" {
            n147 = Bundle By Name(cluster=w394, "4"=w395) -> (w393:T14)
          }
          frame "1" {
            n148 = Bundle By Name(cluster=w397, "1"=w398) -> (w396:T14)
          }
        }
        n149 = Bundle By Name(cluster=w367, "AllNoise"=w363) -> (w360:T1)
      }
      frame "Noise_SumdTrace" {
        # "11:45 pm is 1,425th minute of the day"
        # "Check if it is \"today\". If no, do nothing."
        # "If yes, average the sums and send to Log Loop.\nReset \"today\" value to tomorrow's date."
        # "If no, do nothing."
        # "Check if it is later than 11:45 pm."
        # "Set the date to log. (Today.)"
        # "===Log noise trace at 11:45 pm.==="
        n150 = Unbundle By Name(w452) -> ("AllNoise"=w450:T14, "FPGA.Channel"=w443:T3, "Config.FP_User"=w441:T7)
        n151 = Seconds To Date/Time() -> (date time rec=w437:T23)  [unwired: 2 in]
        n152 = Unbundle By Name(w437) -> ("day of year"=w435:i32, "hour"=w434:i32, "minute"=w431:i32)
        n153 = case shown="\"1\"" w443 {
          tunnel: w450 -> [w498 w502 w506 w510]
          tunnel: [w497 w501 w505 w509] -> w424
          tunnel: w441 -> [w496 w500 w504 w508]
          tunnel: [w495 w499 w503 w507] -> _
          frame "4" {
            n154 = Unbundle By Name(w498) -> ("4"=w497:T15)
            n155 = Unbundle By Name(w496) -> ("4"=w495:T9)
          }
          frame "3" {
            n156 = Unbundle By Name(w502) -> ("3"=w501:T15)
            n157 = Unbundle By Name(w500) -> ("3"=w499:T9)
          }
          frame "2" {
            n158 = Unbundle By Name(w506) -> ("2"=w505:T15)
            n159 = Unbundle By Name(w504) -> ("2"=w503:T9)
          }
          frame "1" {
            n160 = Unbundle By Name(w510) -> ("1"=w509:T15)
            n161 = Unbundle By Name(w508) -> ("1"=w507:T9)
          }
        }
        n162 = Multiply(x=w434, y=60) -> (x*y=w432:i32)
        n163 = Unbundle By Name(w424) -> ("AvgAvgSpectrum"=w447:dbl[], "SumdSpectrum"=w446:dbl[], "SumCount"=w423:u32, "DayOfYear"=w436:i32)
        n164 = Add(x=w432, y=w431) -> (x+y=w428:i32)
        n165 = Greater Or Equal?(x=w428, y=1425) -> (x >= y?=w427:bool)
        n166 = Greater Or Equal?(x=w435, y=w436) -> (x >= y?=w430:bool)
        n167 = call "Sum_Noise_Traces.vi"("SumCount"=w423, "SumdSpectrum"=w446, "AvgAvgSpectrum"=w447) -> ("SumCount"=w422:u32, "SumdSpectrum"=w440:dbl[])  [unwired: 7 in]
        n168 = And(x=w430, y=w427) -> (x .and. y?=w429:bool)
        n169 = case shown="True" w429 {
          tunnel: w445 -> [w456 w480]
          tunnel: [w456 w464] -> w444
          tunnel: w443 -> [_ w475]
          tunnel: w422 -> [w455 w467]
          tunnel: [w455 u32 0] -> w442
          tunnel: w440 -> [w454 w470]
          tunnel: [w454 w469] -> w439
          tunnel: w438 -> [_ w469]
          tunnel: [w453 w460] -> w425
          tunnel: w424 -> [w453 w461]
          frame False {
          }
          frame True {
            # "Average of sums"
            # "At 11:59 pm, send summed array to log loop and change \"day of year\" to tomorrow."
            n170 = To Double Precision Float(number=w467) -> (double precision float=w466:dbl)
            n171 = Divide(x=w470, y=w466) -> (x/y=w468:dbl[])
            n172 = Obtain Queue(name (unnamed)="Log", element data type=cluster{"Enum":T19, "Data":variant} {"Enum"=enum."Log_NoiseTrace", "Data"=variant}, error in (no error)=w480) -> (queue out=w478:refnum<queue>, error out=w479:errorcluster)  [unwired: 2 in, 1 out]
            n173 = Seconds To Date/Time() -> (date time rec=w459:T23)  [unwired: 2 in]
            n174 = Bundle By Name(cluster=cluster{"Target":T3, "NoiseTrace":dbl[]} {"Target"=enum."1", "NoiseTrace"=[]}, "Target"=w475, "NoiseTrace"=w468) -> (w474:cluster{"Target":T3, "NoiseTrace":dbl[]})
            n175 = Unbundle By Name(w459) -> ("day of year"=w458:i32)
            n176 = To Variant(anything=w474) -> (Variant=w473:variant)
            n177 = Increment(x=w458) -> (x+1=w457:i32)
            n178 = Bundle By Name(cluster=cluster{"Enum":T19, "Data":variant} {"Enum"=enum."Log_NoiseTrace", "Data"=variant} ("element"), "Data"=w473) -> (w472:cluster{"Enum":T19, "Data":variant})
            n179 = Bundle By Name(cluster=w461, "DayOfYear"=w457) -> (w460:T15)
            n180 = Enqueue Element(queue=w478, element=w472, timeout in ms (-1)=10, error in (no error)=w479) -> (queue out=w463:refnum<queue>, error out=w465:errorcluster)  [unwired: 1 out]
            n181 = Release Queue(queue=w463, error in (no error)=w465) -> (error out=w464:errorcluster)  [unwired: 1 in, 2 out]
          }
        }
        n182 = Bundle By Name(cluster=w425, "SumdSpectrum"=w439, "SumCount"=w442) -> (w451:T15)
        n183 = case shown="\"4\"" w443 {
          tunnel: w451 -> [w485 w488 w491 w494]
          tunnel: w450 -> [w484 w487 w490 w493]
          tunnel: [w483 w486 w489 w492] -> w449
          frame "2" {
            n184 = Bundle By Name(cluster=w484, "2"=w485) -> (w483:T14)
          }
          frame "3" {
            n185 = Bundle By Name(cluster=w487, "3"=w488) -> (w486:T14)
          }
          frame "4" {
            n186 = Bundle By Name(cluster=w490, "4"=w491) -> (w489:T14)
          }
          frame "1" {
            n187 = Bundle By Name(cluster=w493, "1"=w494) -> (w492:T14)
          }
        }
        n188 = Bundle By Name(cluster=w452, "AllNoise"=w449) -> (w448:T1)
      }
      frame "Noise_Send" {
        # "Reset\nWatchdog"
        # "Only log noise sum every 60 seconds. No averaging."
        # "Send noise data to FP update loop"
        n189 = Unbundle By Name(w540) -> ("FPGA.Channel"=w517:T3, "AllNoise"=w539:T14)
        n190 = call "Watchdog_Functional_Global.vi"("Watchdog"=WatchdogTimer_Enum."Noise", "error in"=w512) -> ("error out"=w511:errorcluster)  [unwired: 7 in, 2 out]
        n191 = case shown="\"1\"" w517 {
          tunnel: w539 -> [w571 w573 w575 w577]
          tunnel: [w570 w572 w574 w576] -> w522
          frame "2" {
            n192 = Unbundle By Name(w571) -> ("2"=w570:T15)
          }
          frame "3" {
            n193 = Unbundle By Name(w573) -> ("3"=w572:T15)
          }
          frame "4" {
            n194 = Unbundle By Name(w575) -> ("4"=w574:T15)
          }
          frame "1" {
            n195 = Unbundle By Name(w577) -> ("1"=w576:T15)
          }
        }
        n196 = Get Date/Time In Seconds() -> (seconds since 1Jan1904=w515:timestamp)
        n197 = Unbundle By Name(w522) -> ("df"=w521:dbl, "Sum"=w520:dbl)
        n198 = To Double Precision Float(number=w515) -> (double precision float=w514:dbl)
        n199 = Bundle By Name(cluster=cluster{"Target":T3, "HDF5_NoiseInfo":T21} {"Target"=enum."1", "HDF5_NoiseInfo"={"Timestring"="Timestamp string goes here", "Timestamp"=0.0, "df"=7629.39453125, "Sum"=0.0}}, "Target"=w517, "HDF5_NoiseInfo.df"=w521, "HDF5_NoiseInfo.Sum"=w520, "HDF5_NoiseInfo.Timestamp"=w514) -> (w525:cluster{"Target":T3, "HDF5_NoiseInfo":T21})
        n200 = Bundle(cluster=cluster{"Target":T3, "1":T15} {"Target"=enum."1", "1"={"df"=0.0, "AvgAvgSpectrum"=[], "FFT_Index"=[], "Avg'd"=[], "Sum"=0.0, "SumdSpectrum"=[], "SumCount"=0, "DayOfYear"=0}}, "Target"=w517, "1"=w522) -> (w538:cluster{"Target":T3, "1":T15})
        n201 = To Variant(anything=w538) -> (Variant=w531:variant)
        n202 = To Variant(anything=w525) -> (Variant=w523:variant)
        n203 = case shown="\"4\"" w517 {
          tunnel: w511 -> [w544 w548 w552 w556]
          tunnel: [w543 w547 w551 w555] -> w519
          tunnel: [w542 w546 w550 w554] -> w518
          frame "1" {
            n204 = call "Elapsed Time4"("Time Target (s)"=60.0, "error in (no error)"=w544) -> ("Time has Elapsed"=w542:bool, "error out"=w543:errorcluster)  [unwired: 10 in, 6 out]
          }
          frame "2" {
            n205 = call "Elapsed Time"("Time Target (s)"=60.0, "error in (no error)"=w548) -> ("Time has Elapsed"=w546:bool, "error out"=w547:errorcluster)  [unwired: 10 in, 6 out]
          }
          frame "3" {
            n206 = call "Elapsed Time2"("Time Target (s)"=60.0, "error in (no error)"=w552) -> ("Time has Elapsed"=w550:bool, "error out"=w551:errorcluster)  [unwired: 10 in, 6 out]
          }
          frame "4" {
            n207 = call "Elapsed Time3"("Time Target (s)"=60.0, "error in (no error)"=w556) -> ("Time has Elapsed"=w554:bool, "error out"=w555:errorcluster)  [unwired: 10 in, 6 out]
          }
        }
        n208 = case shown="True" w518 {
          tunnel: w519 -> [w557 w567]
          tunnel: [w557 w561] -> w530
          tunnel: w523 -> [_ w559]
          frame False {
          }
          frame True {
            n209 = Bundle By Name(cluster=cluster{"Enum":T19, "Data":variant} {"Enum"=enum."Log_NoiseSum", "Data"=variant}, "Data"=w559) -> (w563:cluster{"Enum":T19, "Data":variant})
            n210 = Obtain Queue(max queue size (-1, unlimited)=100, name (unnamed)="Log", element data type=w563, error in (no error)=w567) -> (queue out=w564:refnum<queue>, error out=w565:errorcluster)  [unwired: 1 in, 1 out]
            n211 = Enqueue Element(queue=w564, element=w563, timeout in ms (-1)=10, error in (no error)=w565) -> (queue out=w560:refnum<queue>, error out=w562:errorcluster)  [unwired: 1 out]
            n212 = Release Queue(queue=w560, error in (no error)=w562) -> (error out=w561:errorcluster)  [unwired: 1 in, 2 out]
          }
        }
        n213 = Bundle By Name(cluster=cluster{"Enum":T22, "Data":variant} {"Enum"=enum."FP_Noise", "Data"=variant}, "Data"=w531) -> (w537:cluster{"Enum":T22, "Data":variant})
        n214 = Obtain Queue(max queue size (-1, unlimited)=100, name (unnamed)="FP", element data type=w537, error in (no error)=w530) -> (queue out=w533:refnum<queue>, error out=w534:errorcluster)  [unwired: 1 in, 1 out]
        n215 = Enqueue Element(queue=w533, element=w537, timeout in ms (-1)=10, error in (no error)=w534) -> (queue out=w527:refnum<queue>, error out=w529:errorcluster)  [unwired: 1 out]
        n216 = Release Queue(queue=w527, error in (no error)=w529) -> (error out=w528:errorcluster)  [unwired: 1 in, 2 out]
      }
      frame "Noise_Exit" {
        n217 = Release Queue(queue=w580, error in (no error)=w581) -> (error out=w582:errorcluster)  [unwired: 1 in, 2 out]
      }
    }
    "NoiseLoopCount" <- w11
  }
  "error out" <- w2
